vi "PicoScopeospaGetTimebase.vi"(4 "Number of Samples":u64, 6 "Memory Segment":u64, 7 "Acquisition Settings":T1={"preTriggerSamples"=0, "postTriggerSamples"=1000, "timebase"=2} {"postTriggerSamples" format="%_6p"; "preTriggerSamples" format="%_6p"}, 8 "error in (no error)":errorcluster, 11 "handle in":i16) -> (0 "error out":errorcluster, 3 "handle out":i16, 5 "Properties Panel":T2 {"Max Total Capture Time Available (sec)" format="%.3p"; "Sample Frequency" format="%.6p"; "Sample Rate" format="%.3p"; "Max Samples Available" format="%_6p"; "Total Capture Time (sec)" format="%.3p"})   [LabVIEW 2024]
doc: "Calls Gettimebase function"
uses:
  shared/Acquisition Settings.ctl
  psospa.dll
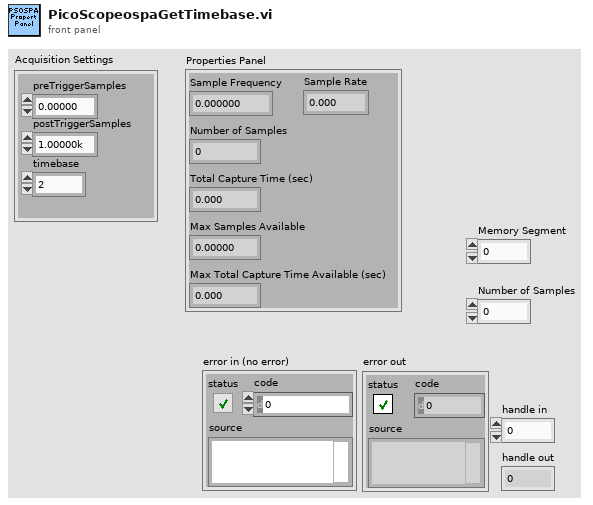
[diagram p1: front panel]
types:
  T1 = typedef "Acquisition Settings.ctl" = cluster{"preTriggerSamples":u64, "postTriggerSamples":u64, "timebase":u32}
  T2 = cluster{"Sample Frequency":dbl, "Sample Rate":dbl, "Max Samples Available":u64, "Number of Samples":u64, "Total Capture Time (sec) ":dbl, "Max Total Capture Time Available (sec)":dbl}
  T3 = cluster{sgl, sgl, "maxSamples":i32, "Number of Samples":u32, sgl, sgl}
  T4 = cluster{"status":bool, "code":u32, "source":string}
  T5 = cluster{dbl, dbl, "maxSamples":u64, "Number of Samples":u64, dbl, dbl}
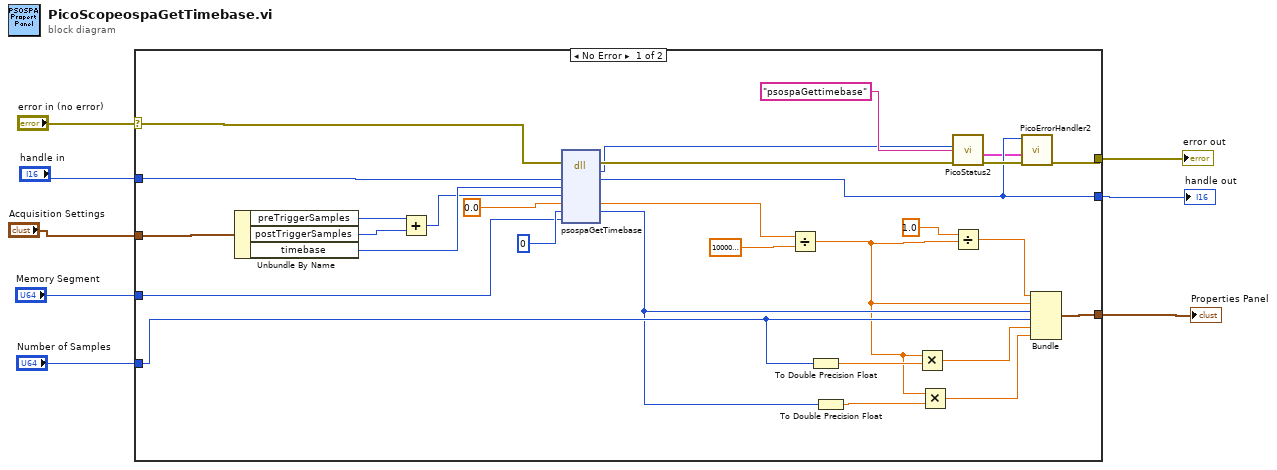
[diagram p0: block diagram]
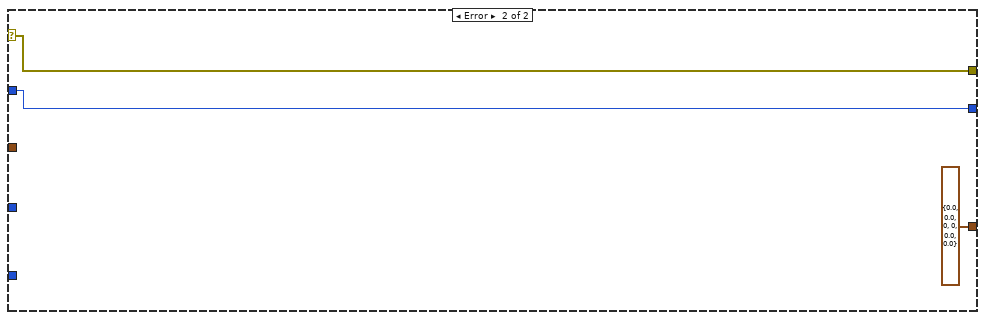
[diagram p2: hidden frame]
diagram:
  n1 = case shown="No Error" "error in (no error)" {
    selector: "error in (no error)" -> [w14 w40]
    tunnel: [w12 w40] -> w8
    tunnel: [w11 w39] -> w7
    tunnel: "Memory Segment" -> [w28 _]
    tunnel: "Number of Samples" -> [w22 _]
    tunnel: "handle in" -> [w27 w39]
    tunnel: "Acquisition Settings" -> [w26 _]
    tunnel: [w18 T3 {0.0, 0.0, "maxSamples"=0, "Number of Samples"=0, 0.0, 0.0}] -> w2
    frame No Error {
      n2 = Unbundle By Name(w26) -> ("preTriggerSamples"=w32:u64, "postTriggerSamples"=w33:u64, "timebase"=w34:u32)
      n3 = Add(x=w32, y=w33) -> (x+y=w24:u64)
      n4 = dll-call lib="F:/Picoscope3000e/Scope_LabView/ps3000e/Treiber_und_SubVis/psospa.dll" fn="psospaGetTimebase"(error in=w14, "handle"=w27, "timebase"=w34, "noSamples"=w24, "timeIntervalNanoseconds"=0.0, "maxSamples"=u64 0, "segmentIndex"=w28) -> (error out=w35:errorcluster, "PICO_STATUS"=w10:u32, "handle"=w11:i16, "timeIntervalNanoseconds"=w36:dbl, "maxSamples"=w20:u64)  [unwired: 5 in, 1 out]
      n5 = Divide(x=w36, y=1000000000.0) -> (x/y=w17:dbl)
      n6 = To Double Precision Float(number=w22) -> (double precision float=w25:dbl)
      n7 = To Double Precision Float(number=w20) -> (double precision float=w21:dbl)
      n8 = Multiply(x=w17, y=w25) -> (x*y=w23:dbl)
      n9 = Multiply(x=w17, y=w21) -> (x*y=w19:dbl)
      n10 = call "PicoStatus2.vi"("PICO source"="psospaGettimebase" ("source"), "Error in"=w35, "PICO STATUS"=w10) -> ("error out"=w13:errorcluster, "PICO_STATUS out"=w9:T4)  [unwired: 5 in]
      n11 = Divide(x=1.0, y=w17) -> (x/y=w15:dbl)
      n12 = call "PicoErrorHandler2.vi"("error in (no error)"=w13, "PICO_STATUS in"=w9, "handle In"=w11) -> ("error out"=w12:errorcluster)  [unwired: 8 in]
      n13 = Bundle(w15, w17, "maxSamples"=w20, "Number of Samples"=w22, w23, w19) -> (w18:T5)  [unwired: 1 in]
    }
    frame Error {
    }
  }
  "error out" <- w8
  "handle out" <- w7
  "Properties Panel" <- w2
